vi "3-and.vi"(1 "Boolean 2":bool, 2 "Boolean 4":bool, 3 "Boolean 3":bool) -> (0 "Boolean":bool)   [LabVIEW 2018]
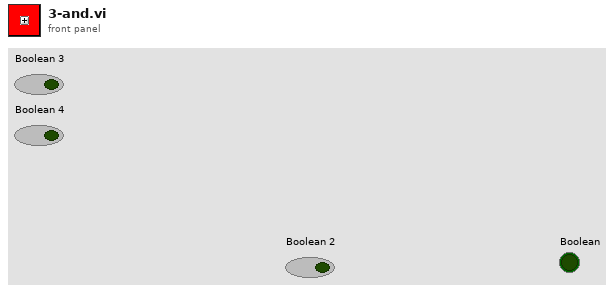
[diagram p1: front panel]
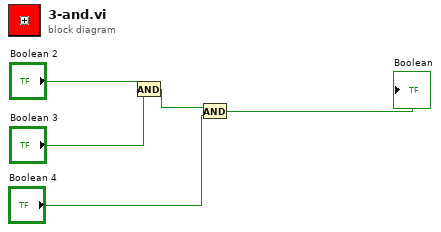
[diagram p0: block diagram]
diagram:
  n1 = And(x="Boolean 2", y="Boolean 3") -> (x .and. y?=w2:bool)
  n2 = And(x=w2, y="Boolean 4") -> (x .and. y?=→"Boolean":bool)
